vi "Build VI.vi"(8 "error in (no error)":errorcluster, 11 "Map":map{string, T1}(c390)) -> (0 "error out":errorcluster)   [LabVIEW 2025]
uses:
  Controls/bd.ctl
  Classes/Node/Node.lvclass
  Controls/wire.ctl
  Controls/Terminal.ctl
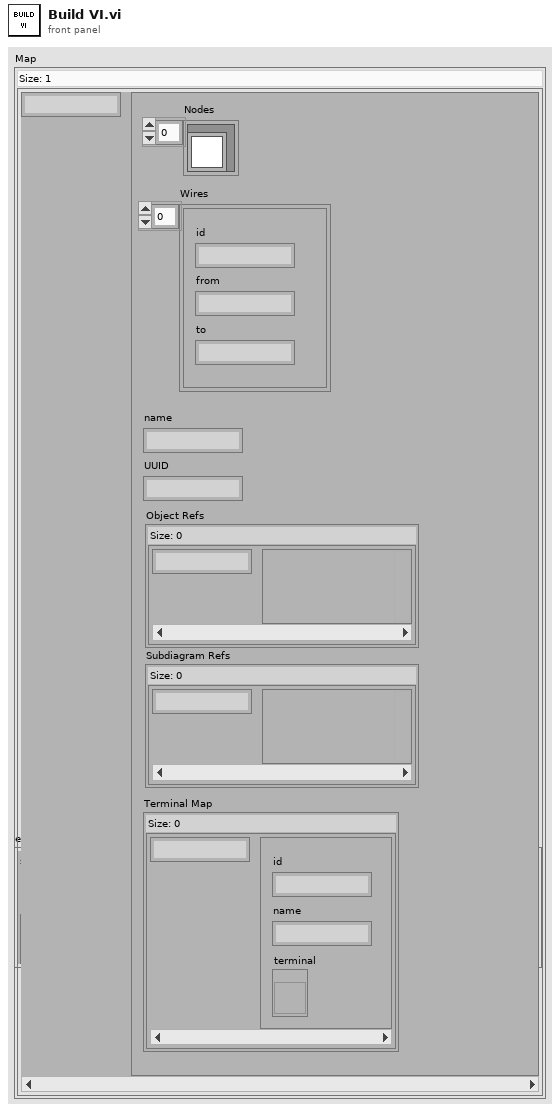
[diagram p1: front panel]
types:
  T1 = typedef "bd.ctl" = cluster{"Nodes":refnum<class "Node.lvclass">[], "Wires":T2[], "name":string, "UUID":string, "Object Refs":map{string, variant}, "Subdiagram Refs":map{string, variant}, "Terminal Map":map{string, T3}}
  T2 = typedef "wire.ctl" = cluster{"id":string, "from":string, "to":string}
  T3 = typedef "Terminal.ctl" = cluster{"id":string, "name":string, "terminal":refnum<vi>}
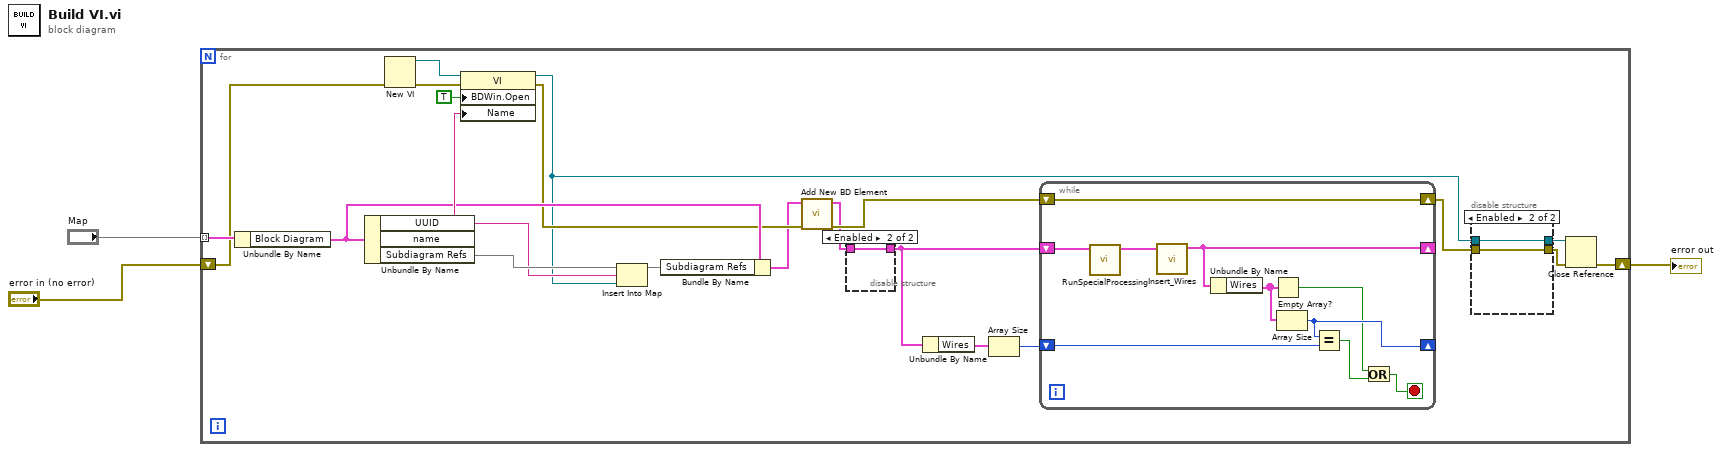
[diagram p0: block diagram]
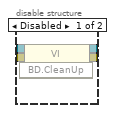
[diagram p2: hidden frame]
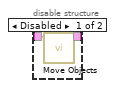
[diagram p3: hidden frame]
diagram:
  n1 = for {
    tunnel: "Map" -> [w25] mode=indexing
    shift-right: [w10] -> w3
    shift-left: "error in (no error)" -> [w14]
    n2 = Unbundle By Name(w25) -> ("Block Diagram"=w20:T1)
    n3 = Unbundle By Name(w20) -> ("UUID"=w6:string, "name"=w21:string, "Subdiagram Refs"=w7:map{string, variant})
    n4 = New VI(8:w14) -> (0:w15:errorcluster, 3:w24:refnum<vi>)  [unwired: 6 in]
    n5 = property class="VI"(reference=w24, error in=w15, "BDWin.Open"=TRUE ("Block Diagram Window:Open"), "Name"=w21) -> (reference out=w5:refnum<vi>, error out=w13:errorcluster)
    n6 = Insert Into Map(map in=w7, key=w6, value=w5) -> (map out=w4:map{string, variant})  [unwired: 2 out]
    n7 = Bundle By Name(cluster=w20, "Subdiagram Refs"=w4) -> (w9:T1)
    n8 = call "Add New BD Element.vi"("error in (no error)"=w13, "Block Diagram in"=w9) -> ("error out"=w12:errorcluster, "Block Diagram out"=w8:T1)  [unwired: 8 in]
    n9 = disable-structure shown="Enabled" {
      disable-tunnel: [w33 w34] -> w19
      disable-tunnel: w8 -> [w32 w34]
      frame Disabled {
        n10 = call "Move Objects.vi"("cluster in"=w32) -> ("cluster out"=w33:T1)  [unwired: 10 in]
      }
      frame Enabled {
      }
    }
    n11 = Unbundle By Name(w19) -> ("Wires"=w18:T2[])
    n12 = Array Size(array=w18) -> (size(s)=w17:i32)
    n13 = while {
      shift-right: [w42] -> _
      shift-left: w19 -> [w44]
      shift-right: [w39] -> _
      shift-left: w17 -> [w40]
      shift-right: [w35] -> w16
      shift-left: w12 -> [w35]
      stop <- w38 stop-if-true
      n14 = call "RunSpecialProcessing.vi"("cluster in"=w44) -> ("cluster out"=w43:T1)  [unwired: 10 in]
      n15 = call "Insert_Wires.vi"("cluster in"=w43) -> ("output cluster"=w42:T1)  [unwired: 10 in]
      n16 = Unbundle By Name(w42) -> ("Wires"=w41:T2[])
      n17 = Empty Array?(array=w41) -> (empty?=w37:bool)
      n18 = Array Size(array=w41) -> (size(s)=w39:i32)
      n19 = Equal?(x=w39, y=w40) -> (x = y?=w36:bool)
      n20 = Or(x=w37, y=w36) -> (x .or. y?=w38:bool)
    }
    n21 = disable-structure shown="Enabled" {
      disable-tunnel: [w29 w31] -> w22
      disable-tunnel: w16 -> [w28 w30]
      disable-tunnel: [w27 w30] -> w11
      disable-tunnel: w5 -> [w26 w31]
      frame Disabled {
        n22 = invoke class="VI" method="BD.CleanUp"(reference=w26, error in=w28) -> (reference out=w29:refnum<vi>, error out=w27:errorcluster)  [unwired: 1 in, 1 out]
      }
      frame Enabled {
      }
    }
    n23 = Close Reference(reference=w22, error in (no error)=w11) -> (error out=w10:errorcluster)
  }
  "error out" <- w3
